vi "Clear IP.vi"(8 "error in (no error)":errorcluster, 11 "APU in":refnum<class "APU.lvclass">) -> (0 "error out":errorcluster)   [LabVIEW 2013, in "APU.lvclass"]
uses:
  APU.lvclass
  Engine Simulation IP.lvclass
  <vilib>/rvi/interface/nirviCloseFPGA/nirviCloseFPGA.xnode
  <vilib>/FPGAPlugInAG/Dynamic/niLvFpga_Close_Dynamic.vi
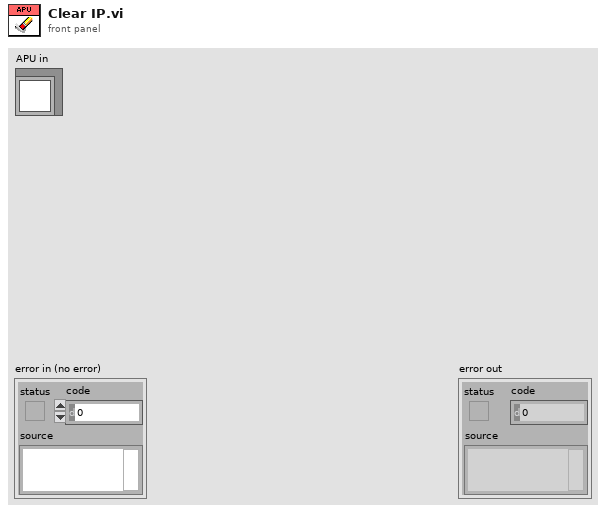
[diagram p1: front panel]
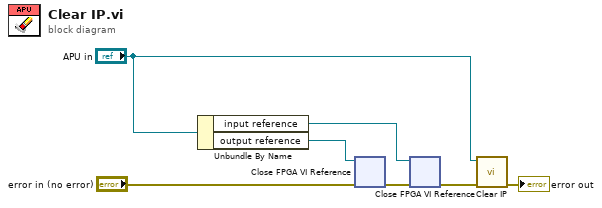
[diagram p0: block diagram]
diagram:
  n1 = Unbundle By Name("APU in") -> ("input reference"=w3:refnum<k20>, "output reference"=w5:refnum<k20>)
  n2 = xnode "Close FPGA VI Reference"("FPGA VI Reference In"=w5, "error in"="error in (no error)") -> ("error out"=w4:errorcluster)
  n3 = xnode "Close FPGA VI Reference"("FPGA VI Reference In"=w3, "error in"=w4) -> ("error out"=w2:errorcluster)
  n4 = call-parent "Clear IP.vi"("error in (no error)"=w2, "Engine Simulation IP in"="APU in") -> ("error out"=→"error out":errorcluster)  [unwired: 9 in]
